vi "PH_Cam_BaseClass.read DB.vi"(0 "DB Entry to read":string, 1 "error in (no error)":errorcluster) -> (2 "Image Type":T1 {"Image Type" items=["Grayscale (U8)", "Grayscale (I16)", "Grayscale (SGL)", "Complex (CSG)", "RGB (U32)", "HSL (U32)", "RGB (U64)", "Grayscale (U16)"]}, 3 "Camera ID":string, 4 "Window Number":i32, 5 "error out":errorcluster)   [LabVIEW 2014, in "PH_Cam_BaseClass.lvlib"]
uses:
  PH_Cam_BaseClass.lvlib
  PH_Cam_BaseClass.Image Type.ctl
  PH_Common/PH_Common.lvlib
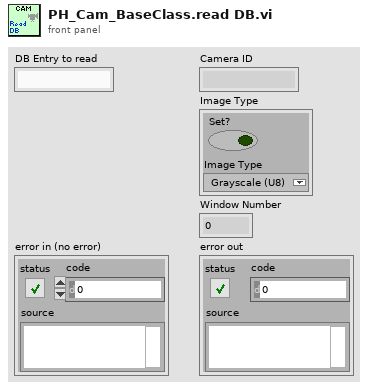
[diagram p1: front panel]
types:
  T1 = typedef "PH_Cam_BaseClass.lvlib/PH_Cam_BaseClass.Image Type.ctl" = cluster{"Set?":bool, "Image Type":T2}
  T2 = typedef "Image Type" = u32
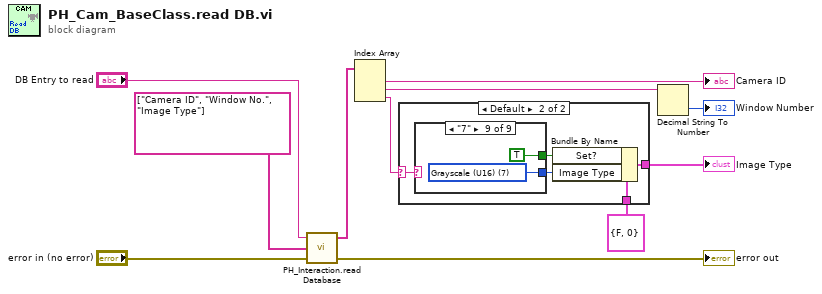
[diagram p0: block diagram]
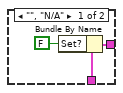
[diagram p2: hidden frame]
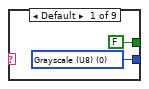
[diagram p3: hidden frame]
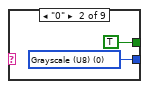
[diagram p4: hidden frame]
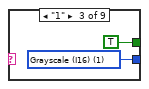
[diagram p5: hidden frame]
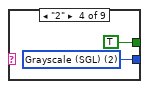
[diagram p6: hidden frame]
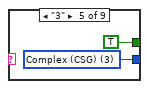
[diagram p7: hidden frame]
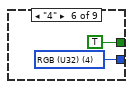
[diagram p8: hidden frame]
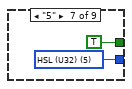
[diagram p9: hidden frame]
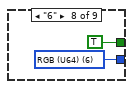
[diagram p10: hidden frame]
diagram:
  n1 = call "PH_Interaction.read Database.vi"("error in (no error)"="error in (no error)", "Strings to search for"=string[] ["Camera ID", "Window No.", "Image Type"] ("Strings to search for in"), "DB Entry to read"="DB Entry to read") -> ("error out"=→"error out":errorcluster, "Values"=w8:string[])  [unwired: 1 in]
  n2 = Index Array(array=w8) -> (element #1=→"Camera ID":string, element #2=w10:string, element #3=w3:string)  [unwired: 3 in]
  n3 = case shown="Default" w3 {
    selector: w3 -> [_ w16]
    tunnel: T1 {"Set?"=FALSE, "Image Type"=0} ("input cluster") -> [w14 w19]
    tunnel: [w13 w18] -> w1
    frame "", "N/A" {
      n4 = Bundle By Name(cluster=w14, "Set?"=FALSE) -> (w13:T1)
    }
    frame Default {
      n5 = case shown="\"7\"" w16 {
        tunnel: [w20 w23 w25 w27 w29 w31 w33 w35 w37] -> w17
        tunnel: [FALSE TRUE TRUE TRUE TRUE TRUE TRUE TRUE TRUE] -> w15
        frame Default {
          w20 = T2 0 items=["Grayscale (U8)", "Grayscale (I16)", "Grayscale (SGL)", "Complex (CSG)", "RGB (U32)", "HSL (U32)", "RGB (U64)", "Grayscale (U16)"] ("Image Type")
        }
        frame "0" {
          w23 = T2 0 items=["Grayscale (U8)", "Grayscale (I16)", "Grayscale (SGL)", "Complex (CSG)", "RGB (U32)", "HSL (U32)", "RGB (U64)", "Grayscale (U16)"] ("Image Type")
        }
        frame "1" {
          w25 = T2 1 items=["Grayscale (U8)", "Grayscale (I16)", "Grayscale (SGL)", "Complex (CSG)", "RGB (U32)", "HSL (U32)", "RGB (U64)", "Grayscale (U16)"] ("Image Type")
        }
        frame "2" {
          w27 = T2 2 items=["Grayscale (U8)", "Grayscale (I16)", "Grayscale (SGL)", "Complex (CSG)", "RGB (U32)", "HSL (U32)", "RGB (U64)", "Grayscale (U16)"] ("Image Type")
        }
        frame "3" {
          w29 = T2 3 items=["Grayscale (U8)", "Grayscale (I16)", "Grayscale (SGL)", "Complex (CSG)", "RGB (U32)", "HSL (U32)", "RGB (U64)", "Grayscale (U16)"] ("Image Type")
        }
        frame "4" {
          w31 = T2 4 items=["Grayscale (U8)", "Grayscale (I16)", "Grayscale (SGL)", "Complex (CSG)", "RGB (U32)", "HSL (U32)", "RGB (U64)", "Grayscale (U16)"] ("Image Type")
        }
        frame "5" {
          w33 = T2 5 items=["Grayscale (U8)", "Grayscale (I16)", "Grayscale (SGL)", "Complex (CSG)", "RGB (U32)", "HSL (U32)", "RGB (U64)", "Grayscale (U16)"] ("Image Type")
        }
        frame "6" {
          w35 = T2 6 items=["Grayscale (U8)", "Grayscale (I16)", "Grayscale (SGL)", "Complex (CSG)", "RGB (U32)", "HSL (U32)", "RGB (U64)", "Grayscale (U16)"] ("Image Type")
        }
        frame "7" {
          w37 = T2 7 items=["Grayscale (U8)", "Grayscale (I16)", "Grayscale (SGL)", "Complex (CSG)", "RGB (U32)", "HSL (U32)", "RGB (U64)", "Grayscale (U16)"] ("Image Type")
        }
      }
      n6 = Bundle By Name(cluster=w19, "Set?"=w15, "Image Type"=w17) -> (w18:T1)
    }
  }
  "Image Type" <- w1
  n7 = Decimal String To Number(string=w10) -> (number=→"Window Number":i32)  [unwired: 2 in, 1 out]
